vi "GEOM_GetHeaders.vi"(8 "error in (no error)":errorcluster, 10 "readmode":string) -> (0 "error out":errorcluster, 1 "S Headers":string[][](array[string]), 2 "ME Headers":string[][][](array[string]))   [LabVIEW 2016]
uses:
  GEOM_VAR_action.ctl
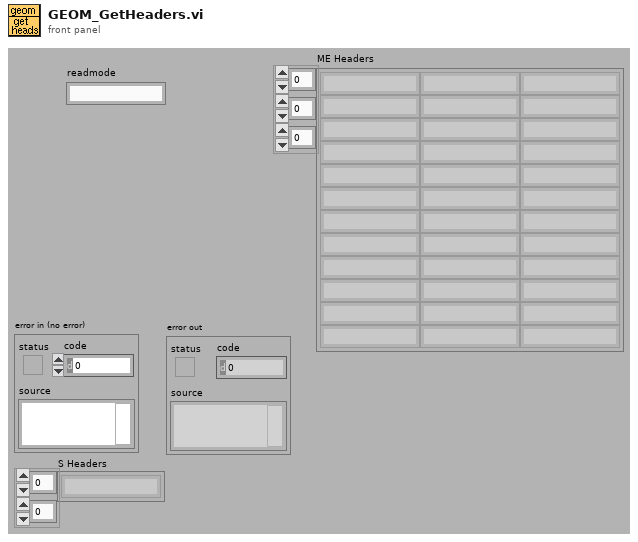
[diagram p1: front panel]
types:
  T1 = typedef "GEOM_VAR_action.ctl" = enum16{"read", "write"}
  T2 = typedef "GEOM_ReadModeHeader.ctl" = cluster{"readmode":string, "ME Headers":string[][][], "S Headers":string[][]}
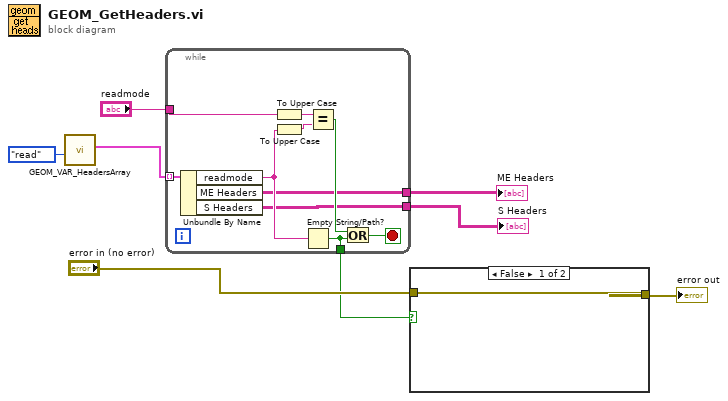
[diagram p0: block diagram]
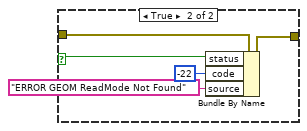
[diagram p2: hidden frame]
diagram:
  n1 = call "GEOM_VAR_HeadersArray.vi"("Action"=GEOM_VAR_action."read") -> ("GEOM_HeadersArray out"=w1:T2[])  [unwired: 1 in, 9 out]
  n2 = while {
    tunnel: "readmode" -> [w18]
    tunnel: w1 -> [w16] mode=indexing
    tunnel: [w11] -> w7
    tunnel: [w10] -> w4
    tunnel: [w9] -> w3
    stop <- w12 stop-if-true
    n3 = Unbundle By Name(w16) -> ("readmode"=w13:string, "ME Headers"=w11:string[][][], "S Headers"=w9:string[][])
    n4 = To Upper Case(1:w18) -> (0:w17:string)
    n5 = To Upper Case(1:w13) -> (0:w15:string)
    n6 = Empty String/Path?(string/path=w13) -> (empty?=w10:bool)
    n7 = Equal?(x=w17, y=w15) -> (x = y?=w14:bool)
    n8 = Or(x=w14, y=w10) -> (x .or. y?=w12:bool)
  }
  "ME Headers" <- w7
  "S Headers" <- w3
  n9 = case shown="False" w4 {
    selector: w4 -> [_ w20]
    tunnel: "error in (no error)" -> [w19 w24]
    tunnel: [w19 w23] -> w5
    frame False {
    }
    frame True {
      n10 = Bundle By Name(cluster=w24, "status"=w20, "code"=-22, "source"="ERROR GEOM ReadMode Not Found") -> (w23:errorcluster)
    }
  }
  "error out" <- w5
